vi "He3ReadOut.vi"(7 "stop_external":refnum<vi>, 10 "status_ref":refnum<vi>, 11 "pressure_ref":refnum<vi>) -> ()   [LabVIEW 2019]
uses:
  <vilib>/Instr/_visa.llb/VISA Flush IO Buffer Mask.ctl
  <vilib>/Utility/config.llb/Read Key (String).vi
  <vilib>/Instr/_visa.llb/VISA Configure Serial Port (Instr).vi
  Global 1.vi
  <vilib>/Utility/config.llb/NI_LVConfig.lvlib
panel:
  out "status string":string
  out "Array":bool[](array[boolean])
  out "Error at VISA Read 6":errorcluster
  out "Error at segmenting output 5":errorcluster
  out "MKS 670 Status":bool
  out "Read buffer":string
  in  "Pressure (Torr)":dbl
  in  "stop":bool
  out "He3 Sensor":dbl
  out "Waveform Chart 2":dbl(graph)
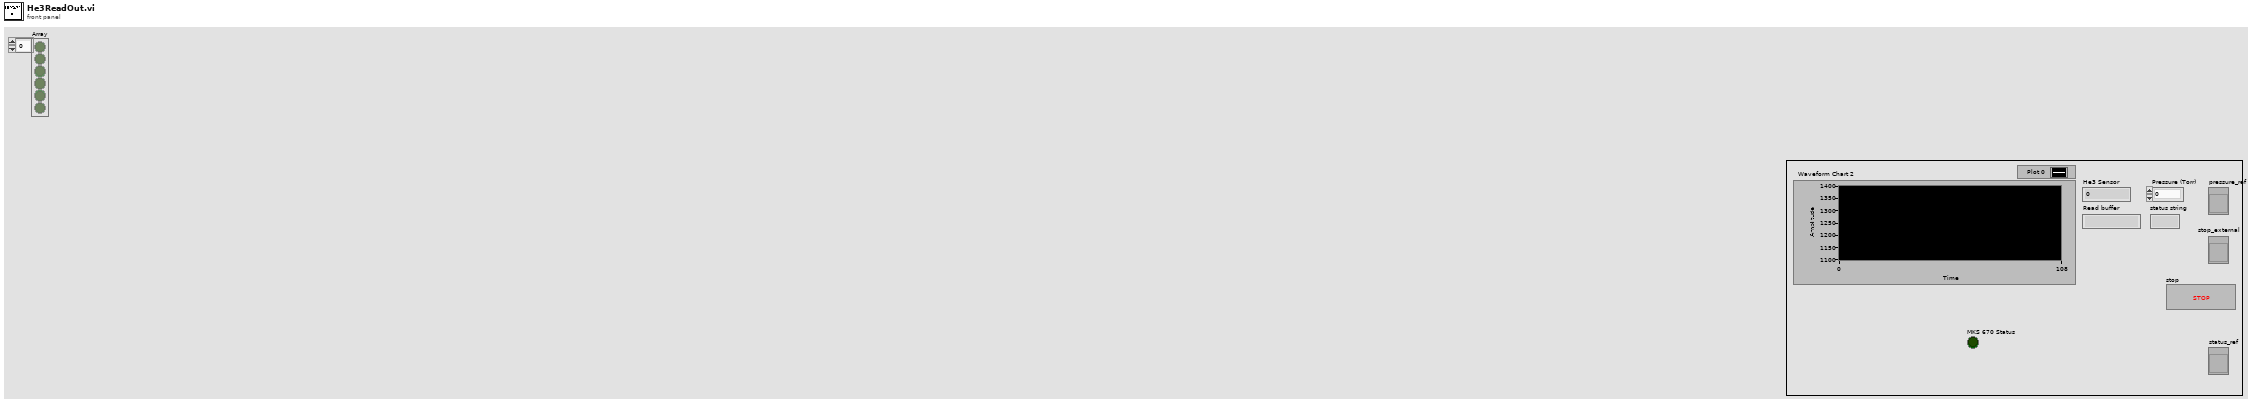
[diagram p1: front panel]
types:
  T1 = typedef "NI_LVConfig.lvlib/Config Data RefNum.ctl" = refnum<k1>
  T2 = typedef "VISA Flush IO Buffer Mask.ctl" = u16
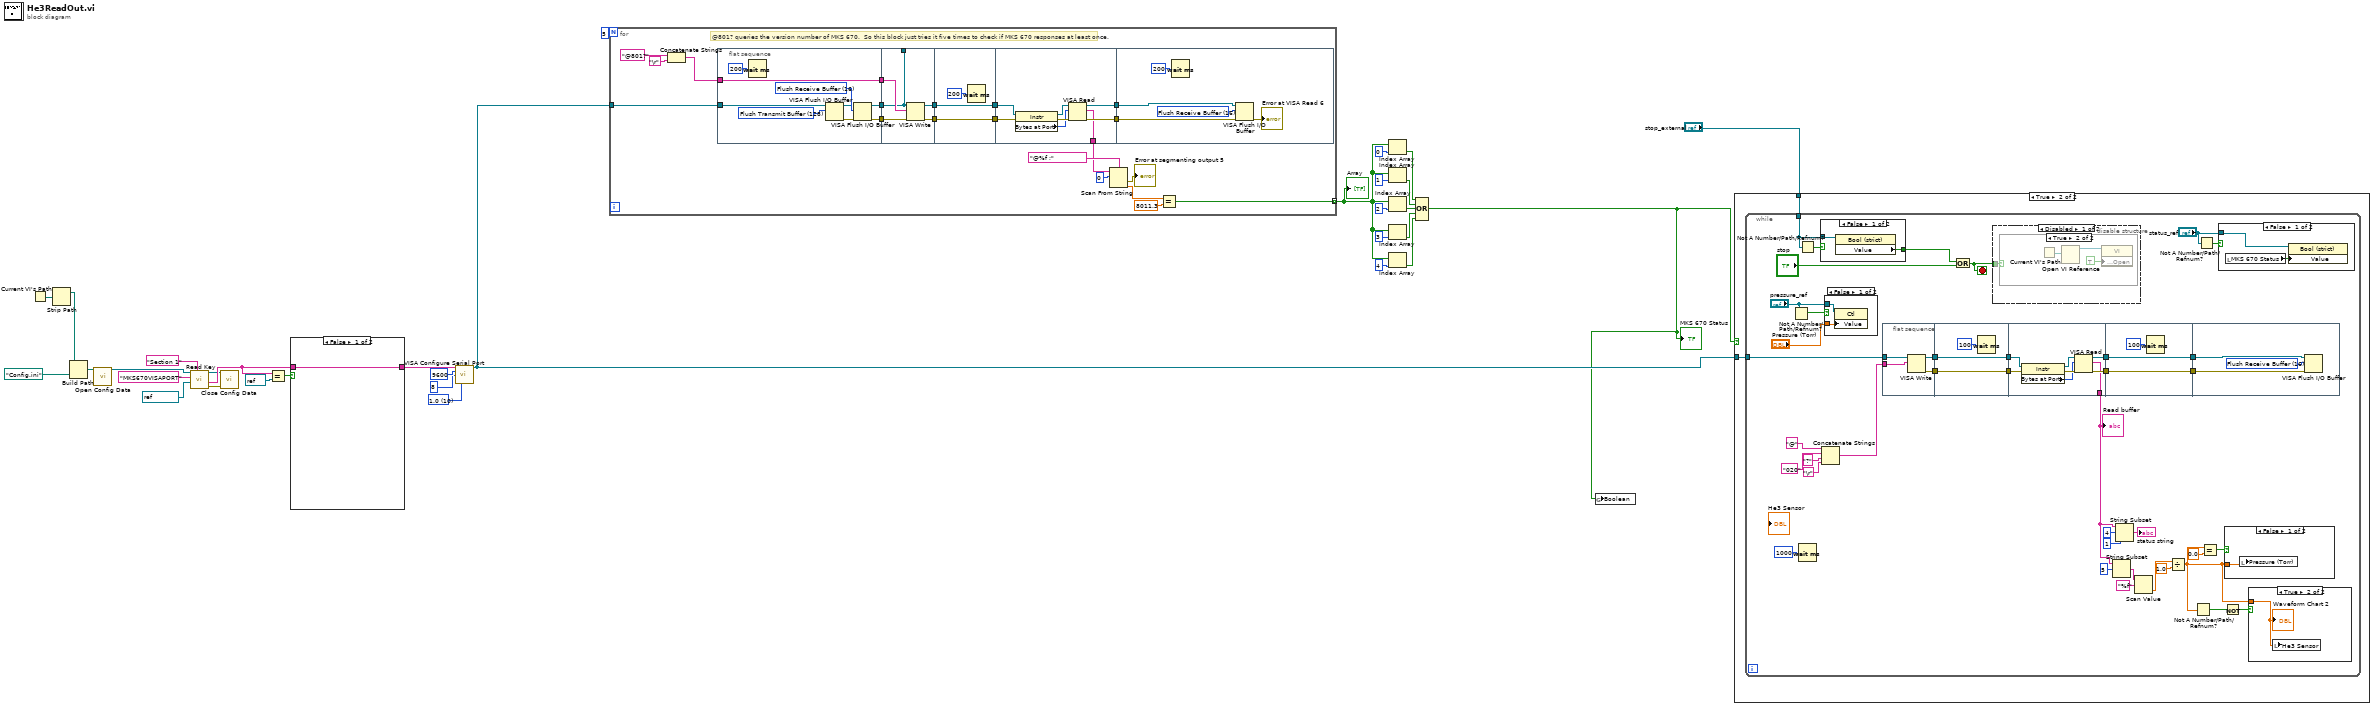
[diagram p0: block diagram]
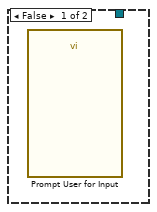
[diagram p2: hidden frame]
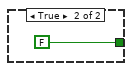
[diagram p7: hidden frame]
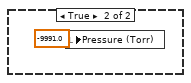
[diagram p8: hidden frame]
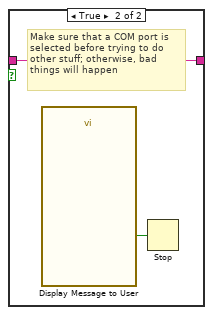
[diagram p10: hidden frame]
diagram:
  w21 = u16 10 items=["1.0"=10, "1.5"=15, "2.0"=20] ("stop bits (10: 1 bit)")
  n1 = Current VI's Path() -> (path=w4:path)
  n2 = Strip Path(path=w4) -> (stripped path=w3:path)  [unwired: 1 out]
  n3 = Build Path(base path=w3, name or relative path=path "Config.ini" ("default name")) -> (appended path=w29:path)
  n4 = call <vilib>:"Open Config Data.vi"("configuration file path"=w29) -> ("refnum"=w24:T1)  [unwired: 8 in, 2 out]
  n5 = call-poly <vilib>:"Read Key.vi"("section"="Section 1", "default value"=refnum<visa-resource-name> "COM1" ("VISA resource name"), "key"="MKS670VISAPORT", "refnum"=w24) -> ("error out"=w30:errorcluster, "value"=w32:string, "refnum out"=w26:T1)  [unwired: 4 in, 1 out]
  n6 = call <vilib>:"Close Config Data.vi"("error in (no error)"=w30, "refnum"=w26) -> ()  [unwired: 8 in, 2 out]
  n7 = Equal?(x=w32, y=refnum<visa-resource-name> refnum) -> (x = y?=w22:bool)
  n8 = case shown="False" w22 {
    tunnel: [w33 w34] -> w18
    tunnel: w32 -> [w33 w34]
    frame False {
    }
    frame True {
      # "Make sure that a COM port is\nselected before trying to do\nother stuff; otherwise, bad\nthings will happen"
      n9 = call "Display Message to User"() -> ("Got it, thanks"=w35:bool)  [unwired: 10 in, 1 out]
      n10 = Stop(stop? (T)=w35) -> ()
    }
  }
  n11 = call-poly "VISA Configure Serial Port"("VISA resource name"=w18, "baud rate (9600)"=u32 9600, "data bits (8)"=u16 8, "stop bits (10: 1 bit)"=w21) -> ("VISA resource name out"=w5:refnum<visa-resource-name>)  [unwired: 10 in, 1 out]
  n12 = for {
    N: 5 -> [_]
    tunnel: w5 -> [w40]
    tunnel: [w39] -> w6 mode=indexing
    # "@801? queries the version number of MKS 670.  So this block just tries it five times to check if MKS 670 responses at least once."
    n13 = Concatenate Strings("@801?" ("string"), "\r") -> (w36:string)
    n14 = flat-sequence {
      tunnel: w40 -> [w59]
      tunnel: w36 -> [w64]
      tunnel: [w64] -> w55
      tunnel: [w58] -> w54
      tunnel: [w57] -> w53
      tunnel: [w66] -> _
      tunnel: [w68] -> w52
      tunnel: [w67] -> w51
      tunnel: w55 -> [w69]
      tunnel: w54 -> [w66]
      tunnel: w53 -> [w65]
      tunnel: w52 -> [w71]
      tunnel: [w71] -> w50
      tunnel: w51 -> [w70]
      tunnel: [w70] -> w49
      tunnel: w50 -> [w77]
      tunnel: w49 -> [w76]
      tunnel: [w75] -> w48
      tunnel: [w74] -> w47
      tunnel: [w73] -> w41
      tunnel: w48 -> [w84]
      tunnel: w47 -> [w83]
      frame #0 {
        w63 = T2 16 items=["Flush Receive Buffer"=16, "Write Transmit Buffer to Device"=32, "Flush Receive Buffer (No I/O)"=64, "Flush Transmit Buffer"=128] ("Mask")
        w60 = T2 128 items=["Flush Receive Buffer"=16, "Write Transmit Buffer to Device"=32, "Flush Receive Buffer (No I/O)"=64, "Flush Transmit Buffer"=128] ("Mask")
        n15 = Wait (ms)(milliseconds to wait=u32 200) -> ()  [unwired: 1 out]
        n16 = VISA Flush I/O Buffer(VISA resource name=w59, mask (16)=w60) -> (VISA resource name out=w61:refnum<visa-resource-name>, error out=w62:errorcluster)  [unwired: 1 in]
        n17 = VISA Flush I/O Buffer(VISA resource name=w61, mask (16)=w63, error in (no error)=w62) -> (VISA resource name out=w58:refnum<visa-resource-name>, error out=w57:errorcluster)
      }
      frame #1 {
        n18 = VISA Write(VISA resource name=w66, write buffer=w69, error in (no error)=w65) -> (VISA resource name out=w68:refnum<visa-resource-name>, error out=w67:errorcluster)  [unwired: 1 out]
      }
      frame #2 {
        n19 = Wait (ms)(milliseconds to wait=u32 200) -> ()  [unwired: 1 out]
      }
      frame #3 {
        n20 = property class="Instr"(reference=w77, error in=w76) -> (reference out=w78:refnum<visa-resource-name>, error out=w80:errorcluster, "Bytes at Port"=w79:u32)
        n21 = VISA Read(VISA resource name=w78, byte count=w79, error in (no error)=w80) -> (VISA resource name out=w75:refnum<visa-resource-name>, read buffer=w73:string, error out=w74:errorcluster)  [unwired: 1 out]
      }
      frame #4 {
        w81 = T2 16 items=["Flush Receive Buffer"=16, "Write Transmit Buffer to Device"=32, "Flush Receive Buffer (No I/O)"=64, "Flush Transmit Buffer"=128] ("Mask")
        n22 = Wait (ms)(milliseconds to wait=u32 200) -> ()  [unwired: 1 out]
        n23 = VISA Flush I/O Buffer(VISA resource name=w84, mask (16)=w81, error in (no error)=w83) -> (error out=→"Error at VISA Read 6":errorcluster)  [unwired: 1 out]
      }
    }
    n24 = Scan From String(format string="@%f ;", input string=w41, initial scan location=u32 0) -> (error out=→"Error at segmenting output 5":errorcluster, output 1=w43:dbl)  [unwired: 2 in, 2 out]
    n25 = Equal?(x=w43, y=8011.3) -> (x = y?=w39:bool)
  }
  "Array" <- w6
  n26 = Index Array(array=w6, index=0) -> (element=w10:bool)
  n27 = Index Array(array=w6, index=1) -> (element=w11:bool)
  n28 = Index Array(array=w6, index=2) -> (element=w9:bool)
  n29 = Index Array(array=w6, index=3) -> (element=w8:bool)
  n30 = Index Array(array=w6, index=4) -> (element=w7:bool)
  n31 = Compound Arithmetic op=OR(w10, w11, w9, w8, w7) -> (w2:bool)
  "MKS 670 Status" <- w2
  n32 = global write "Global 1.vi" "Boolean"(w2) -> ()
  n33 = case shown="True" w2 {
    tunnel: w5 -> [_ w87]
    tunnel: "stop_external" -> [_ w86]
    frame False {
      n34 = call "Prompt User for Input"() -> ()  [unwired: 18 in, 2 out]
    }
    frame True {
      n35 = while {
        tunnel: w87 -> [w106]
        tunnel: w86 -> [w93]
        stop <- w96 stop-if-true
        n36 = Not A Number/Path/Refnum?(number/path/refnum="pressure_ref") -> (NaN/Path/Refnum?=w88:bool)
        n37 = Not A Number/Path/Refnum?(number/path/refnum=w93) -> (NaN/Path/Refnum?=w97:bool)
        n38 = Wait (ms)(milliseconds to wait=u32 1000) -> ()  [unwired: 1 out]
        n39 = case shown="False" w97 {
          tunnel: [w135 FALSE] -> w94
          tunnel: w93 -> [w136 _]
          frame False {
            n40 = property class="Bool (strict)"(reference=w136) -> ("Value"=w135:bool)  [unwired: 1 in, 2 out]
          }
          frame True {
          }
        }
        n41 = Concatenate Strings("@" ("string"), "020" ("string"), "?" ("string"), "\r") -> (w111:string)
        n42 = case shown="False" w88 {
          tunnel: "pressure_ref" -> [w132 _]
          tunnel: "Pressure (Torr)" -> [w131 _]
          frame False {
            n43 = property class="Ctl"(reference=w132, "Value"=w131) -> ()  [unwired: 1 in, 2 out]
          }
          frame True {
          }
        }
        n44 = flat-sequence {
          tunnel: w111 -> [w141]
          tunnel: w106 -> [w140]
          tunnel: [w139] -> w115
          tunnel: [w138] -> w114
          tunnel: w115 -> [w143]
          tunnel: [w143] -> w113
          tunnel: w114 -> [w142]
          tunnel: [w142] -> w112
          tunnel: w113 -> [w149]
          tunnel: w112 -> [w148]
          tunnel: [w147] -> w110
          tunnel: [w146] -> w109
          tunnel: [w145] -> w101
          tunnel: w110 -> [w155]
          tunnel: w109 -> [w154]
          tunnel: [w155] -> w108
          tunnel: [w154] -> w107
          tunnel: w108 -> [w158]
          tunnel: w107 -> [w157]
          frame #0 {
            n45 = VISA Write(VISA resource name=w140, write buffer=w141) -> (VISA resource name out=w139:refnum<visa-resource-name>, error out=w138:errorcluster)  [unwired: 1 in, 1 out]
          }
          frame #1 {
            n46 = Wait (ms)(milliseconds to wait=u32 100) -> ()  [unwired: 1 out]
          }
          frame #2 {
            n47 = property class="Instr"(reference=w149, error in=w148) -> (reference out=w150:refnum<visa-resource-name>, error out=w152:errorcluster, "Bytes at Port"=w151:u32)
            n48 = VISA Read(VISA resource name=w150, byte count=w151, error in (no error)=w152) -> (VISA resource name out=w147:refnum<visa-resource-name>, read buffer=w145:string, error out=w146:errorcluster)  [unwired: 1 out]
          }
          frame #3 {
            n49 = Wait (ms)(milliseconds to wait=u32 100) -> ()  [unwired: 1 out]
          }
          frame #4 {
            w156 = T2 16 items=["Flush Receive Buffer"=16, "Write Transmit Buffer to Device"=32, "Flush Receive Buffer (No I/O)"=64, "Flush Transmit Buffer"=128] ("Mask")
            n50 = VISA Flush I/O Buffer(VISA resource name=w158, mask (16)=w156, error in (no error)=w157) -> ()  [unwired: 2 out]
          }
        }
        n51 = Or(x=w94, y="stop") -> (x .or. y?=w96:bool)
        n52 = disable-structure shown="Disabled" {
          disable-tunnel: w96 -> [w127 _]
          frame Disabled {
            n53 = case shown="True" w127 {
              frame False {
              }
              frame True {
                n54 = Current VI's Path() -> (path=w130:path)
                n55 = Open VI Reference(vi path=w130) -> (vi reference=w129:refnum<vi>)  [unwired: 5 in, 1 out]
                n56 = property class="VI"(reference=w129, "Front Panel Window:Open"=TRUE) -> ()  [unwired: 1 in, 2 out]
              }
            }
          }
          frame Enabled {
          }
        }
        n57 = String Subset(string=w101, offset (0)=5) -> (substring=w100:string)  [unwired: 1 in]
        n58 = String Subset(string=w101, offset (0)=4, length (rest)=1 ("length (rest)")) -> (substring=→"status string":string)
        n59 = Scan Value(string=w100, format string="%f") -> (value=w98:dbl)  [unwired: 1 in, 1 out]
        n60 = Divide(x=w98, y=1.0) -> (x/y=w116:dbl)
        n61 = Not A Number/Path/Refnum?(number/path/refnum=w116) -> (NaN/Path/Refnum?=w123:bool)
        n62 = Not A Number/Path/Refnum?(number/path/refnum="status_ref") -> (NaN/Path/Refnum?=w92:bool)
        n63 = Equal?(x=w116, y=0.0) -> (x = y?=w117:bool)
        n64 = case shown="False" w92 {
          tunnel: "status_ref" -> [w133 _]
          frame False {
            n65 = local read "MKS 670 Status"() -> (w134:bool)
            n66 = property class="Bool (strict)"(reference=w133, "Value"=w134) -> ()  [unwired: 1 in, 2 out]
          }
          frame True {
          }
        }
        n67 = Not(x=w123) -> (.not. x?=w122:bool)
        n68 = case shown="False" w117 {
          tunnel: w116 -> [w159 _]
          frame False {
            n69 = local write "Pressure (Torr)"(w159) -> ()
          }
          frame True {
            n70 = local write "Pressure (Torr)"(-9991.0 ("Numeric")) -> ()
          }
        }
        n71 = case shown="True" w122 {
          tunnel: w116 -> [_ w161]
          frame False {
          }
          frame True {
            n72 = local write "He3 Sensor"(w161) -> ()
            "Waveform Chart 2" <- w161
          }
        }
        "Read buffer" <- w101
      }
    }
  }
